vi "Fuel v1.2.vi"(1 "INDICATOR INPUT":dbl[](array[numeric]), 2 "BUTTON INPUT":dbl[](array[numeric]), 3 "DATA INPUT":dbl[](array[numeric])) -> (0 "OUTPUT":dbl[](array[numeric]))   [LabVIEW 2019]
uses:
  <vilib>/ptbypt/NI_PtbyPt.lvlib
panel:
  out "PH LED 6":bool=TRUE
  in  "PH CHECK 6":bool
  out "PH IND 6":bool=TRUE
  out "PH LED 5":bool=TRUE
  out "PH LED 4":bool=TRUE
  out "PH LED 3":bool=TRUE
  out "PH LED 2":bool=TRUE
  out "PH LED 1":bool=TRUE
  in  "PH CHECK 1":bool
  in  "PH CHECK 2":bool
  in  "PH CHECK 3":bool
  in  "PH CHECK 4":bool
  in  "PH CHECK 5":bool
  out "PH IND 5":bool=TRUE
  out "PH IND 4":bool=TRUE
  out "PH IND 3":bool=TRUE
  out "PH IND 2":bool=TRUE
  out "PH IND 1":bool=TRUE
  out "IGN TRIP GNG":bool=TRUE
  out "IGN TRIP GNG NUM":dbl
  out "IGN TRIP GNG LED":bool=TRUE
  out "STARTUP GNG":bool=TRUE
  out "STARTUP GNG NUM":dbl
  out "STARTUP GNG LED":bool=TRUE
  out "PURGE GNG":bool=TRUE
  out "PURGE GNG NUM":dbl
  out "PURGE GNG LED":bool=TRUE
  out "RECORD GNG":bool=TRUE
  out "RECORD GNG NUM":dbl
  out "RECORD GNG LED":bool=TRUE
  out "FU VENT GNG":bool=TRUE
  out "FU VENT GNG NUM":dbl
  out "FU VENT GNG LED":bool=TRUE
  out "FU ISO GNG":bool=TRUE
  out "FU ISO GNG NUM":dbl
  out "FU ISO GNG LED":bool=TRUE
  out "OX TANK TEMP 1":dbl
  out "TANK TEMP FU":u32(colorbox)
  out "SUB PANELS GNG":bool=TRUE
  out "SUB PANEL FU GNG NUM":dbl
  out "SUB PANEL FU GNG LED":bool=TRUE
  out "VALVE STATES GNG":bool=TRUE
  out "VALVE ST FU GNG NUM":dbl
  out "VALVE ST FU GNG LED":bool=TRUE
  out "PRESS VALVES GNG":bool=TRUE
  out "PRESS VALVE FU GNG NUM":dbl
  out "PRESS VALVE FU GNG LED":bool=TRUE
  out "ARM GNG":bool=TRUE
  out "ARMED GNG NUM":dbl
  out "ARMED GNG LED":bool=TRUE
  in  "FUEL GNG BUTTON":bool
  out "FU GNG MAIN LED":bool=TRUE
  in  "ABORT BUTTON":bool
  out "ARMED PANEL LED":bool
  out "IGN INSERTED PANEL LED":bool
  out "NANNY PAN LED":bool
  out "SYS STATUS MAIN STRING":string
  out "REG PRESS GNG":bool=TRUE
  out "RELIEF GNG":bool=TRUE
  out "REG PRESS FU GNG NUM":dbl
  out "REG PRESS FU GNG LED":bool=TRUE
  out "RELIEF FU GNG NUM":dbl
  out "RELIEF FU GNG LED":bool=TRUE
  out "TANK PRESS GNG":bool=TRUE
  out "TANK PRESS FU GNG NUM":dbl
  out "TANK PRESS FU GNG LED":bool=TRUE
  out "FILL VALVES GNG":bool=TRUE
  out "FILL VALVE FU GNG NUM":dbl
  out "FILL VALVE FU GNG LED":bool=TRUE
  out "TANK LEVEL GNG":bool=TRUE
  out "TANK LEVEL FU GNG NUM":dbl
  out "TANK LEVEL FU GNG LED":bool=TRUE
  out "FUEL MAIN VALVE TEMP":dbl(slide) scale=-200.0..75.0
  out "FUEL MAIN LINE TEMP":dbl(slide) scale=-200.0..75.0
  out "FUEL VENTURI TEMP":dbl(slide) scale=-200.0..75.0
  out "FUEL TANK RELIEF TEMP":dbl(slide) scale=-200.0..75.0
  out "FUEL TANK TEMP":dbl(slide) scale=-200.0..75.0
  out "MAIN PRESS FU METER":dbl(knob) scale=0.0..1600.0
  out "MAIN LINE PRESS FU METER":dbl(knob) scale=0.0..1600.0
  out "TANK PRESS FU METER":dbl(knob) scale=0.0..1600.0
  out "REG PRESS FU METER":dbl(knob) scale=0.0..1600.0
  out "FUEL SYSTEM PRESSURE":dbl[](graph) caption="Waveform Chart - dark"
  out "FUEL TANK LEVEL (%)":dbl(slide) scale=0.0..100.0
  in  "FUEL FILL BUTTON":bool
  out "FUEL FILL LED":bool=TRUE
  in  "ABV-FU-340 (FUEL PURGE)":bool
  out "ABV-FU-340 LED":bool=TRUE
  in  "ABV-FU-330 (FUEL MAIN)":bool
  out "ABV-FU-330 LED":bool=TRUE
  in  "ABV-FU-320 (FUEL ISO)":bool
  out "ABV-FU-320 LED":bool=TRUE
  in  "ABV-FU-310 (FUEL VENT)":bool
  out "ABV-FU-310 LED":bool=TRUE
  in  "ABV-PR-120 (FUEL PRESS)":bool
  out "ABV-PR-120 LED":bool=TRUE
  # "FUEL CONTROL"
  # "NANNY"
  # "IGNITOR \nINSERTED"
  # "ARMED"
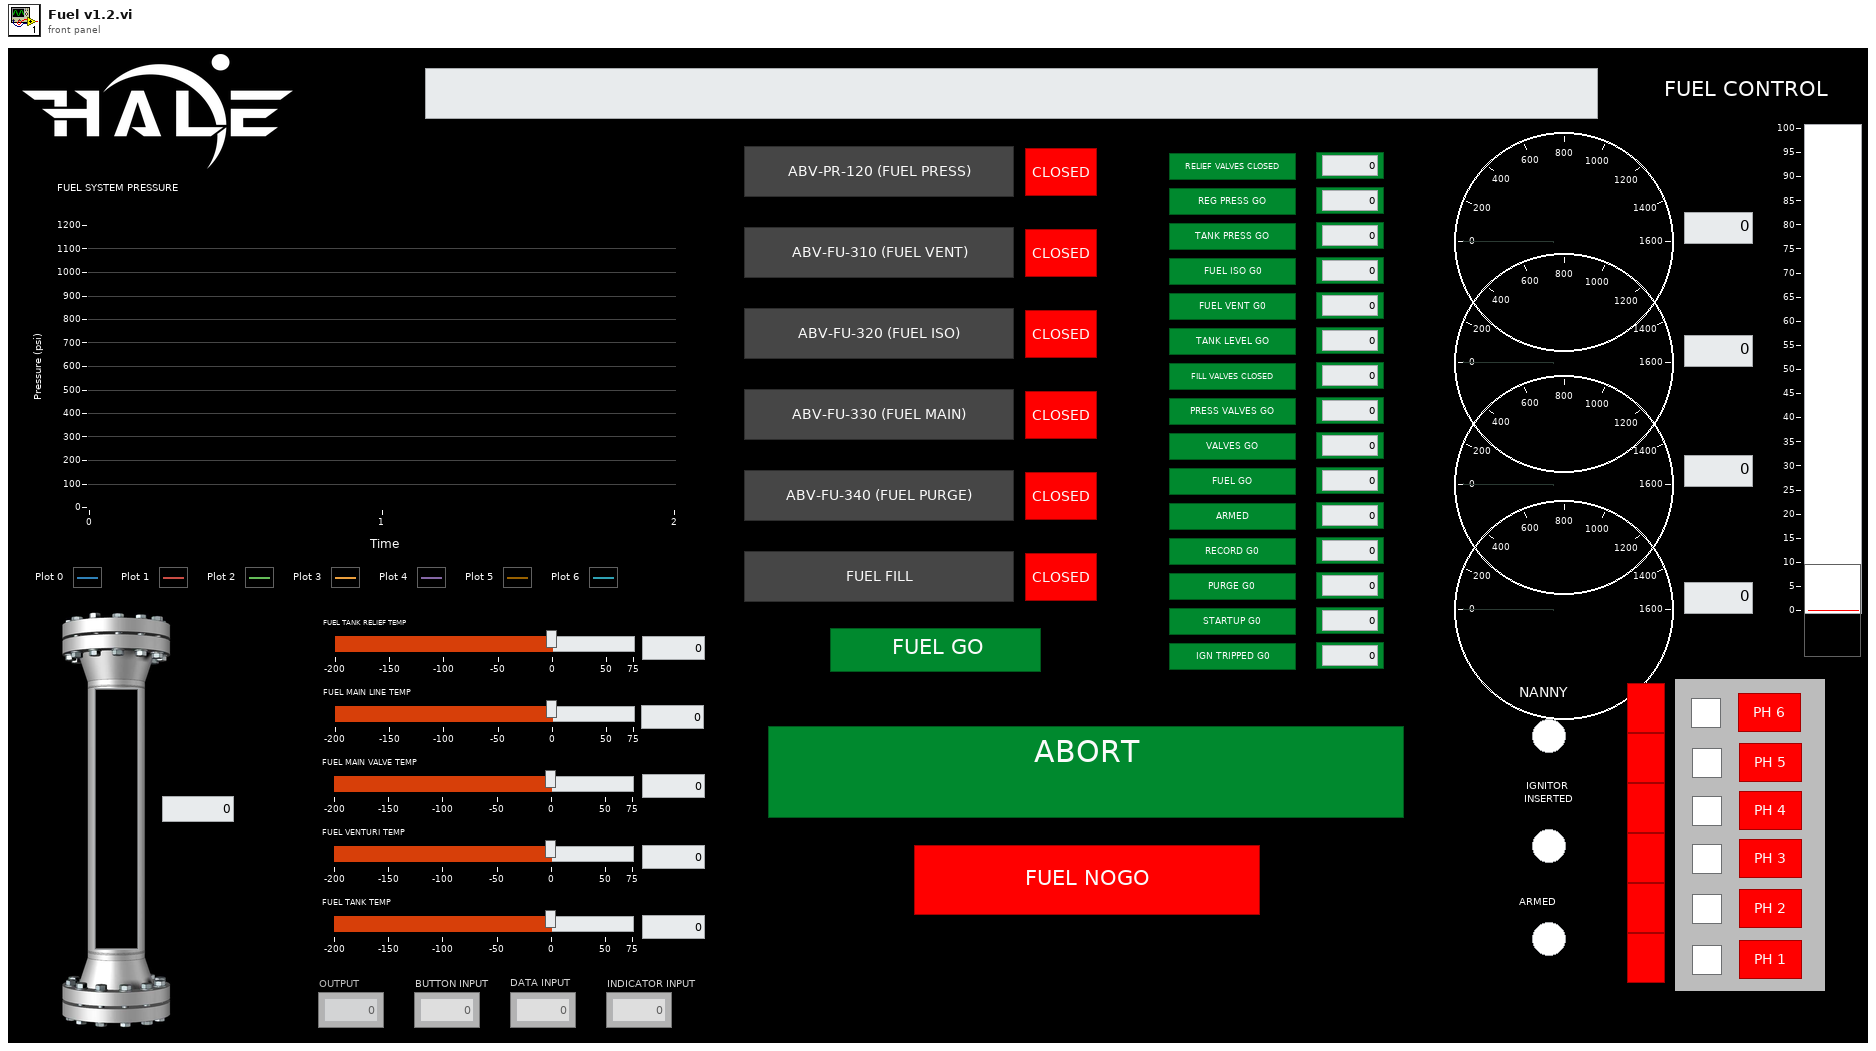
[diagram p1: front panel]
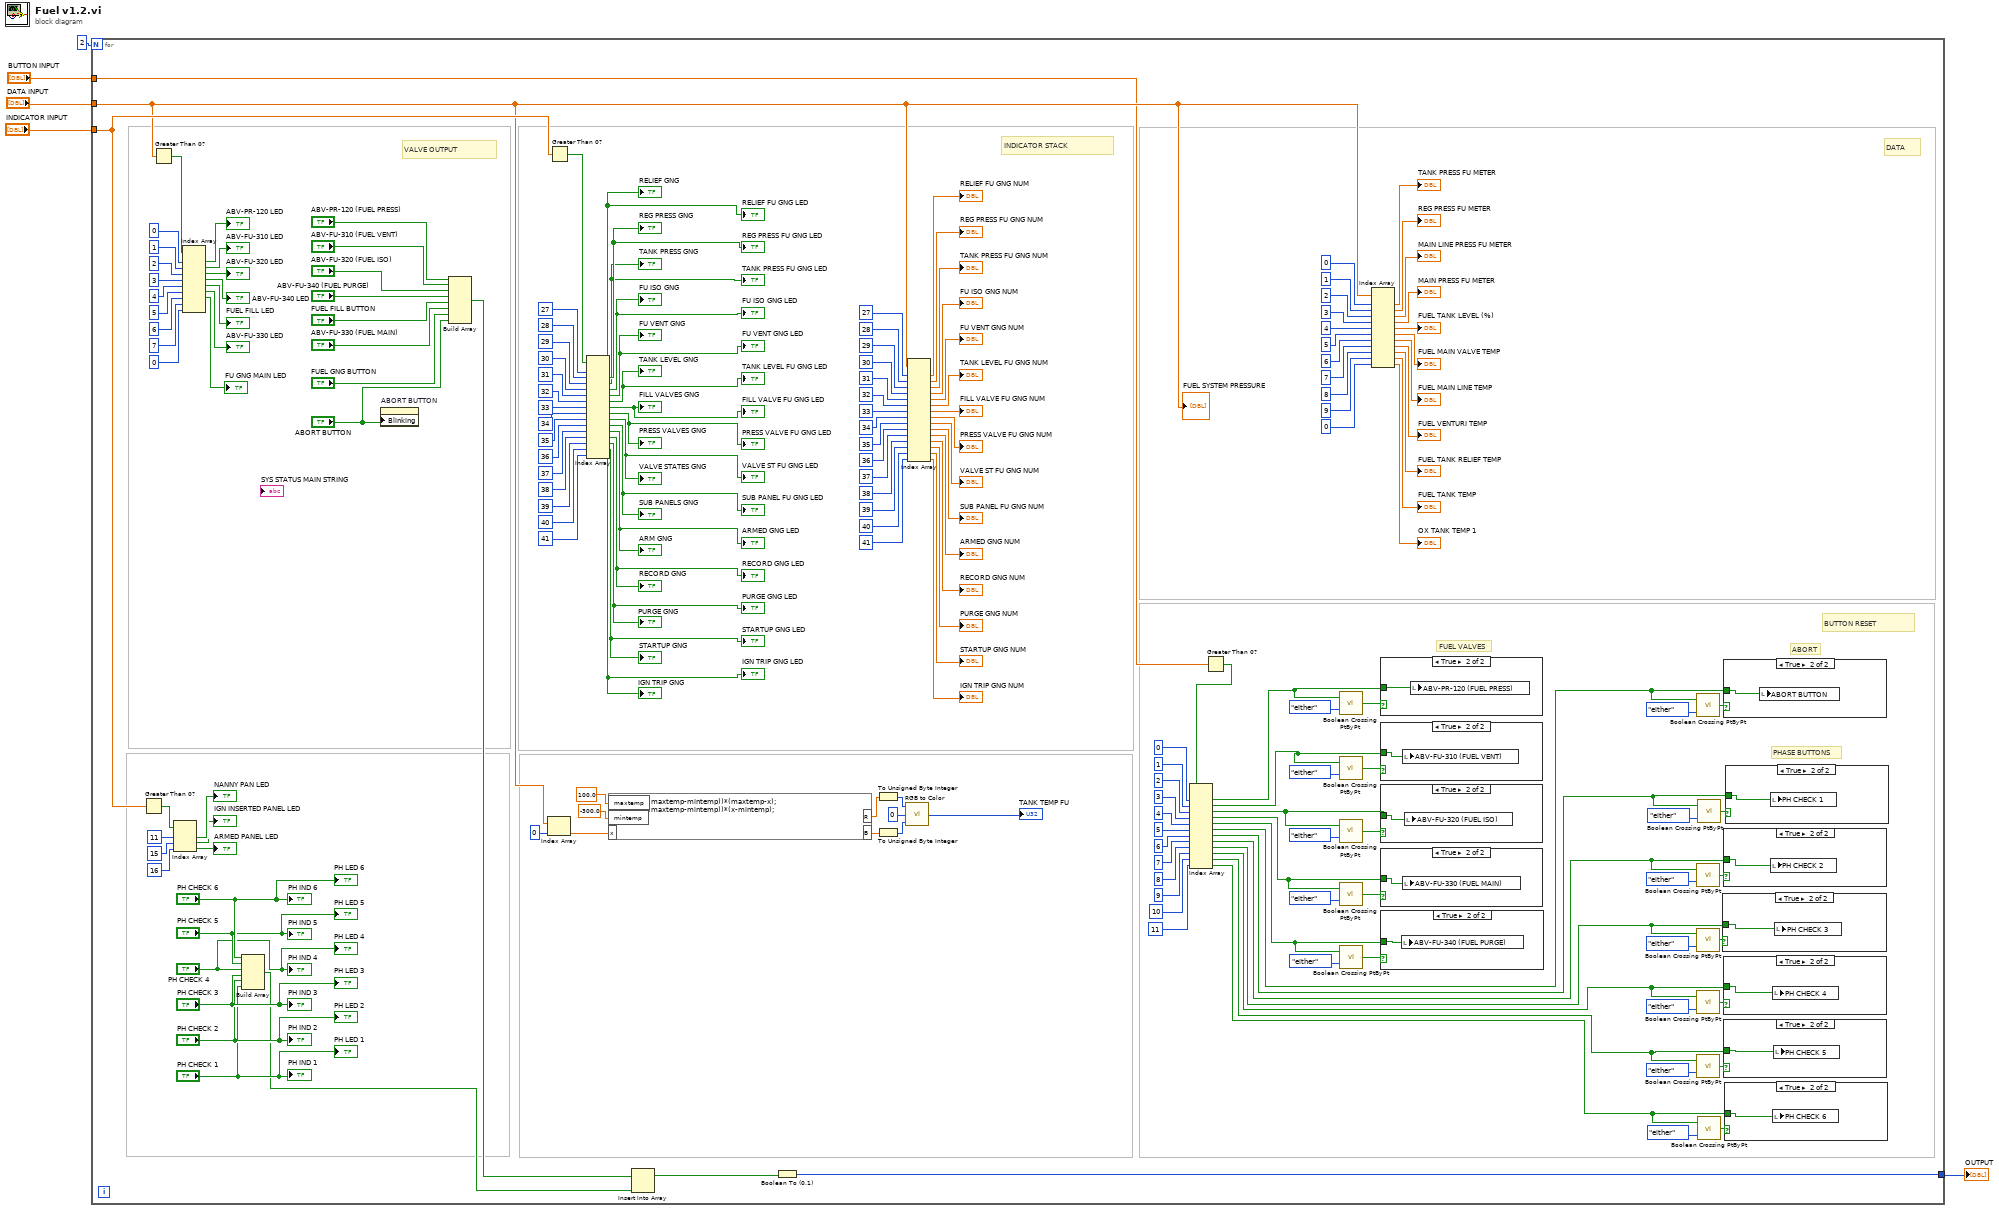
[diagram p0: block diagram]
diagram:
  n1 = for {
    N: 2 -> [_]
    tunnel: "INDICATOR INPUT" -> [w70]
    tunnel: [w69] -> w2
    tunnel: "DATA INPUT" -> [w10]
    tunnel: "BUTTON INPUT" -> [w6]
    # "VALVE OUTPUT"
    # "INDICATOR STACK"
    # "DATA"
    # "BUTTON RESET"
    # "PHASE BUTTONS"
    # "ABORT"
    # "FUEL VALVES"
    n2 = Greater Than 0?(x=w70) -> (x > 0?=w71:bool[])
    n3 = Greater Than 0?(x=w10) -> (x > 0?=w123:bool[])
    n4 = Index Array(array=w71, index #1=11 ("index"), index #2=15 ("index"), index #3=16 ("index")) -> (element #1=→"NANNY PAN LED":bool, element #2=→"IGN INSERTED PANEL LED":bool, element #3=→"ARMED PANEL LED":bool)
    n5 = Index Array(array=w123, index #1=0 ("index"), index #2=1 ("index"), index #3=2 ("index"), index #4=3 ("index"), index #5=4 ("index"), index #6=5 ("index"), index #7=6 ("index"), index #8=7 ("index"), index #9=0 ("index")) -> (element #1=→"ABV-PR-120 LED":bool, element #2=→"ABV-FU-310 LED":bool, element #3=→"ABV-FU-320 LED":bool, element #4=→"ABV-FU-340 LED":bool, element #5=→"FUEL FILL LED":bool, element #6=→"ABV-FU-330 LED":bool, element #7=→"FU GNG MAIN LED":bool)  [unwired: 2 out]
    n6 = Build Array("PH CHECK 6", "PH CHECK 5", "PH CHECK 4", "PH CHECK 3", "PH CHECK 2", "PH CHECK 1") -> (w8:bool[])
    n7 = property on="ABORT BUTTON" class="Bool (strict)"("Blinking"="ABORT BUTTON") -> ()  [unwired: 2 in, 2 out]
    n8 = Build Array("ABV-PR-120 (FUEL PRESS)", "ABV-FU-310 (FUEL VENT)", "ABV-FU-320 (FUEL ISO)", "ABV-FU-340 (FUEL PURGE)", "FUEL FILL BUTTON", "ABV-FU-330 (FUEL MAIN)", "FUEL GNG BUTTON", "ABORT BUTTON") -> (w9:bool[])
    n9 = Index Array(array=w10, index=0) -> (element=w112:dbl)
    n10 = Greater Than 0?(x=w70) -> (x > 0?=w106:bool[])
    n11 = Index Array(array=w106, index #1=27 ("index"), index #2=28 ("index"), index #3=29 ("index"), index #4=30 ("index"), index #5=31 ("index"), index #6=32 ("index"), index #7=33 ("index"), index #8=34 ("index"), index #9=35 ("index"), index #10=36 ("index"), index #11=37 ("index"), index #12=38 ("index"), index #13=39 ("index"), index #14=40 ("index"), index #15=41 ("index")) -> (element #1=→"RELIEF FU GNG LED" →"RELIEF GNG":bool, element #2=→"REG PRESS FU GNG LED" →"REG PRESS GNG":bool, element #3=→"TANK PRESS FU GNG LED" →"TANK PRESS GNG":bool, element #4=→"FU ISO GNG LED" →"FU ISO GNG":bool, element #5=→"FU VENT GNG LED" →"FU VENT GNG":bool, element #6=→"TANK LEVEL FU GNG LED" →"TANK LEVEL GNG":bool, element #7=→"FILL VALVE FU GNG LED" →"FILL VALVES GNG":bool, element #8=→"PRESS VALVE FU GNG LED" →"PRESS VALVES GNG":bool, element #9=→"VALVE ST FU GNG LED" →"VALVE STATES GNG":bool, element #10=→"SUB PANEL FU GNG LED" →"SUB PANELS GNG":bool, element #11=→"ARMED GNG LED" →"ARM GNG":bool, element #12=→"RECORD GNG LED" →"RECORD GNG":bool, element #13=→"PURGE GNG LED" →"PURGE GNG":bool, element #14=→"STARTUP GNG LED" →"STARTUP GNG":bool, element #15=→"IGN TRIP GNG LED" →"IGN TRIP GNG":bool)
    n12 = formula code="B = (255/(maxtemp-mintemp))*(maxtemp-x);\nR = (255/(maxtemp-mintemp))*(x-mintemp);"("maxtemp"=100.0 ("input variable"), "mintemp"=-300.0 ("input variable"), "x"=w112) -> ("B"=w115:dbl, "R"=w117:dbl)
    n13 = Insert Into Array(array=w9, new element=w8) -> (w7:bool[])  [unwired: 1 in]
    n14 = Boolean To (0,1)(Boolean=w7) -> (0, 1=w69:i16[])
    n15 = To Unsigned Byte Integer(number=w117) -> (unsigned 8bit integer=w116:u8)
    n16 = To Unsigned Byte Integer(number=w115) -> (unsigned 8bit integer=w114:u8)
    n17 = call <vilib>:"RGB to Color.vi"("B"=w114, "G"=u8 0, "R"=w116) -> ("Color"=→"TANK TEMP FU":u32)
    n18 = Index Array(array=w10, index #1=27 ("index"), index #2=28 ("index"), index #3=29 ("index"), index #4=30 ("index"), index #5=31 ("index"), index #6=32 ("index"), index #7=33 ("index"), index #8=34 ("index"), index #9=35 ("index"), index #10=36 ("index"), index #11=37 ("index"), index #12=38 ("index"), index #13=39 ("index"), index #14=40 ("index"), index #15=41 ("index")) -> (element #1=→"RELIEF FU GNG NUM":dbl, element #2=→"REG PRESS FU GNG NUM":dbl, element #3=→"TANK PRESS FU GNG NUM":dbl, element #4=→"FU ISO GNG NUM":dbl, element #5=→"FU VENT GNG NUM":dbl, element #6=→"TANK LEVEL FU GNG NUM":dbl, element #7=→"FILL VALVE FU GNG NUM":dbl, element #8=→"PRESS VALVE FU GNG NUM":dbl, element #9=→"VALVE ST FU GNG NUM":dbl, element #10=→"SUB PANEL FU GNG NUM":dbl, element #11=→"ARMED GNG NUM":dbl, element #12=→"RECORD GNG NUM":dbl, element #13=→"PURGE GNG NUM":dbl, element #14=→"STARTUP GNG NUM":dbl, element #15=→"IGN TRIP GNG NUM":dbl)
    n19 = Greater Than 0?(x=w6) -> (x > 0?=w11:bool[])
    n20 = Index Array(array=w11, index #1=0 ("index"), index #2=1 ("index"), index #3=2 ("index"), index #4=3 ("index"), index #5=4 ("index"), index #6=5 ("index"), index #7=6 ("index"), index #8=7 ("index"), index #9=8 ("index"), index #10=9 ("index"), index #11=10 ("index"), index #12=11 ("index")) -> (element #1=w24:bool, element #2=w23:bool, element #3=w22:bool, element #4=w21:bool, element #5=w20:bool, element #6=w19:bool, element #7=w18:bool, element #8=w17:bool, element #9=w16:bool, element #10=w15:bool, element #11=w13:bool, element #12=w12:bool)
    n21 = call <vilib>:"Boolean Crossing PtByPt.vi"("direction"=enum16{"either", "false-true", "true-false"}."either", "input"=w24) -> ("crossing"=w59:bool)  [unwired: 1 in]
    n22 = call <vilib>:"Boolean Crossing PtByPt.vi"("direction"=enum16{"either", "false-true", "true-false"}."either", "input"=w23) -> ("crossing"=w57:bool)  [unwired: 1 in]
    n23 = call <vilib>:"Boolean Crossing PtByPt.vi"("direction"=enum16{"either", "false-true", "true-false"}."either", "input"=w22) -> ("crossing"=w55:bool)  [unwired: 1 in]
    n24 = call <vilib>:"Boolean Crossing PtByPt.vi"("direction"=enum16{"either", "false-true", "true-false"}."either", "input"=w21) -> ("crossing"=w53:bool)  [unwired: 1 in]
    n25 = call <vilib>:"Boolean Crossing PtByPt.vi"("direction"=enum16{"either", "false-true", "true-false"}."either", "input"=w20) -> ("crossing"=w51:bool)  [unwired: 1 in]
    n26 = Index Array(array=w10, index #1=0 ("index"), index #2=1 ("index"), index #3=2 ("index"), index #4=3 ("index"), index #5=4 ("index"), index #6=5 ("index"), index #7=6 ("index"), index #8=7 ("index"), index #9=8 ("index"), index #10=9 ("index"), index #11=0 ("index")) -> (element #1=→"TANK PRESS FU METER":dbl, element #2=→"REG PRESS FU METER":dbl, element #3=→"MAIN LINE PRESS FU METER":dbl, element #4=→"MAIN PRESS FU METER":dbl, element #5=→"FUEL TANK LEVEL (%)":dbl, element #6=→"FUEL MAIN VALVE TEMP":dbl, element #7=→"FUEL MAIN LINE TEMP":dbl, element #8=→"FUEL VENTURI TEMP":dbl, element #9=→"FUEL TANK RELIEF TEMP":dbl, element #10=→"FUEL TANK TEMP":dbl, element #11=→"OX TANK TEMP 1":dbl)
    n27 = case shown="True" w57 {
      tunnel: w23 -> [_ w203]
      frame False {
      }
      frame True {
        n28 = local write "ABV-FU-310 (FUEL VENT)"(w203) -> ()
      }
    }
    n29 = case shown="True" w55 {
      tunnel: w22 -> [_ w202]
      frame False {
      }
      frame True {
        n30 = local write "ABV-FU-320 (FUEL ISO)"(w202) -> ()
      }
    }
    n31 = case shown="True" w53 {
      tunnel: w21 -> [_ w201]
      frame False {
      }
      frame True {
        n32 = local write "ABV-FU-330 (FUEL MAIN)"(w201) -> ()
      }
    }
    n33 = case shown="True" w59 {
      tunnel: w24 -> [_ w204]
      frame False {
      }
      frame True {
        n34 = local write "ABV-PR-120 (FUEL PRESS)"(w204) -> ()
      }
    }
    n35 = case shown="True" w51 {
      tunnel: w20 -> [_ w200]
      frame False {
      }
      frame True {
        n36 = local write "ABV-FU-340 (FUEL PURGE)"(w200) -> ()
      }
    }
    n37 = call <vilib>:"Boolean Crossing PtByPt.vi"("direction"=enum16{"either", "false-true", "true-false"}."either", "input"=w19) -> ("crossing"=w49:bool)  [unwired: 1 in]
    n38 = call <vilib>:"Boolean Crossing PtByPt.vi"("direction"=enum16{"either", "false-true", "true-false"}."either", "input"=w17) -> ("crossing"=w45:bool)  [unwired: 1 in]
    n39 = call <vilib>:"Boolean Crossing PtByPt.vi"("direction"=enum16{"either", "false-true", "true-false"}."either", "input"=w16) -> ("crossing"=w43:bool)  [unwired: 1 in]
    n40 = call <vilib>:"Boolean Crossing PtByPt.vi"("direction"=enum16{"either", "false-true", "true-false"}."either", "input"=w15) -> ("crossing"=w41:bool)  [unwired: 1 in]
    n41 = call <vilib>:"Boolean Crossing PtByPt.vi"("direction"=enum16{"either", "false-true", "true-false"}."either", "input"=w13) -> ("crossing"=w39:bool)  [unwired: 1 in]
    n42 = call <vilib>:"Boolean Crossing PtByPt.vi"("direction"=enum16{"either", "false-true", "true-false"}."either", "input"=w12) -> ("crossing"=w37:bool)  [unwired: 1 in]
    n43 = call <vilib>:"Boolean Crossing PtByPt.vi"("direction"=enum16{"either", "false-true", "true-false"}."either", "input"=w18) -> ("crossing"=w47:bool)  [unwired: 1 in]
    n44 = case shown="True" w43 {
      tunnel: w16 -> [_ w196]
      frame False {
      }
      frame True {
        n45 = local write "PH CHECK 3"(w196) -> ()
      }
    }
    n46 = case shown="True" w49 {
      tunnel: w19 -> [_ w199]
      frame False {
      }
      frame True {
        n47 = local write "ABORT BUTTON"(w199) -> ()
      }
    }
    n48 = case shown="True" w45 {
      tunnel: w17 -> [_ w197]
      frame False {
      }
      frame True {
        n49 = local write "PH CHECK 2"(w197) -> ()
      }
    }
    n50 = case shown="True" w41 {
      tunnel: w15 -> [_ w195]
      frame False {
      }
      frame True {
        n51 = local write "PH CHECK 4"(w195) -> ()
      }
    }
    n52 = case shown="True" w39 {
      tunnel: w13 -> [_ w194]
      frame False {
      }
      frame True {
        n53 = local write "PH CHECK 5"(w194) -> ()
      }
    }
    n54 = case shown="True" w37 {
      tunnel: w12 -> [_ w193]
      frame False {
      }
      frame True {
        n55 = local write "PH CHECK 6"(w193) -> ()
      }
    }
    n56 = case shown="True" w47 {
      tunnel: w18 -> [_ w198]
      frame False {
      }
      frame True {
        n57 = local write "PH CHECK 1"(w198) -> ()
      }
    }
    "FUEL SYSTEM PRESSURE" <- w10
    "PH IND 1" <- "PH CHECK 1"
    "PH IND 2" <- "PH CHECK 2"
    "PH IND 3" <- "PH CHECK 3"
    "PH IND 4" <- "PH CHECK 4"
    "PH IND 5" <- "PH CHECK 5"
    "PH LED 1" <- "PH CHECK 1"
    "PH LED 2" <- "PH CHECK 2"
    "PH LED 3" <- "PH CHECK 3"
    "PH LED 4" <- "PH CHECK 4"
    "PH LED 5" <- "PH CHECK 5"
    "PH LED 6" <- "PH CHECK 6"
    "PH IND 6" <- "PH CHECK 6"
  }
  "OUTPUT" <- w2
